vi "Configure User Margin.vi"(8 "error in (no error)":errorcluster, 9 "User Margin (0)":dbl format="%^.3e", 10 "Instance (1)":T1=1, 11 "VISA resource name":refnum<visa-resource-name>) -> (0 "error out":errorcluster, 3 "VISA resource name out":refnum<visa-resource-name>)   [LabVIEW 2020, in "Rohde&Schwarz CMWXP NR FR1 Measurement.lvlib"]
doc: "Sets the margin that the measurement adds to the expected nominal power to determine the reference power. The reference power minus the external input attenuation must be within the power range of the selected input connector. Refer to the data sheet.\n\nAttribute:\nRSCMWXPNRFR1M_ATTR_USER_MARGIN\n\nRemote-control command:\nCONFigure:NRSub:MEAS<i>:RFSettings:UMARgin"
uses:
  <instrlib>/Rohde&Schwarz CMWXP NR FR1 Measurement/Rohde&Schwarz CMWXP NR FR1 Measurement.lvlib
  <instrlib>/Rohde&Schwarz CMWXP NR FR1 Measurement/Private/_Instance.ctl
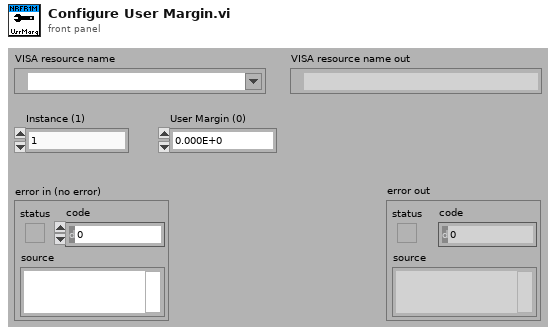
[diagram p1: front panel]
types:
  T1 = typedef "Rohde&Schwarz CMWXP NR FR1 Measurement.lvlib/_Instance.ctl" = i32
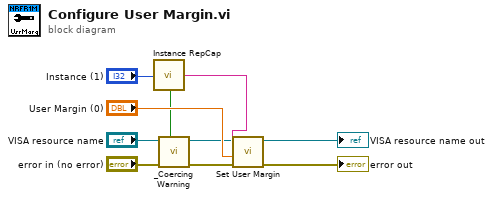
[diagram p0: block diagram]
diagram:
  n1 = call <instrlib>:"Instance RepCap.vi"("Instance In"="Instance (1)") -> ("In Range?"=w1:bool, "RepCap Identifier Out"=w6:string)  [unwired: 1 in]
  n2 = call <instrlib>:"_Coercing Warning.vi"("In Range?"=w1, "error in (no error)"="error in (no error)", "VISA resource name"="VISA resource name") -> ("error out"=w3:errorcluster, "VISA resource name out"=w2:refnum<visa-resource-name>)  [unwired: 7 in]
  n3 = call "Set User Margin"("Repeated Capabilities"=w6, "error in (no error)"=w3, "User Margin (0.0)"="User Margin (0)", "instrument handle"=w2) -> ("error out"=→"error out":errorcluster, "instrument handle out"=→"VISA resource name out":refnum<visa-resource-name>)  [unwired: 6 in]
